vi "Open Front Panel.vi"(8 "Error In":errorcluster, 11 "Display Panel V3 in":refnum<class "Display Panel V3.lvclass">) -> (0 "Error Out":errorcluster, 3 "Display Panel V3 out":refnum<class "Display Panel V3.lvclass">)   [LabVIEW 2014, in "Display Panel.lvlib" / "Display Panel V3.lvclass"]
uses:
  Display Panel V3.lvclass
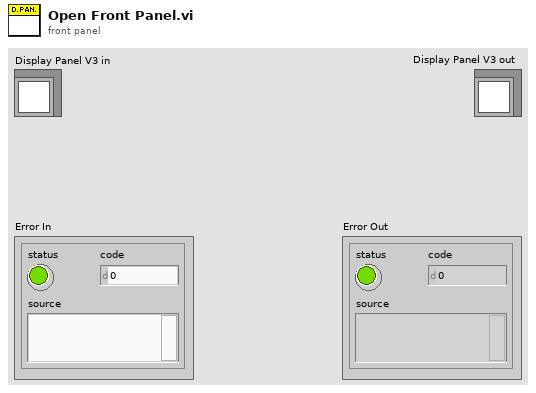
[diagram p1: front panel]
types:
  T1 = enum32{"Invalid", "Standard", "Closed", "Hidden", "Minimized", "Maximized"}
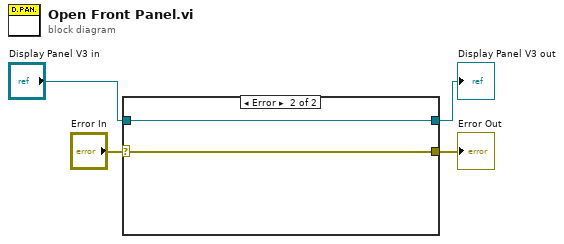
[diagram p0: block diagram]
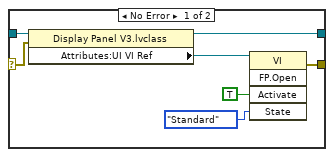
[diagram p2: hidden frame]
diagram:
  n1 = case shown="Error" "Error In" {
    selector: "Error In" -> [w10 w12]
    tunnel: "Display Panel V3 in" -> [w11 w13]
    tunnel: [w6 w12] -> w2
    tunnel: [w5 w13] -> w1
    frame No Error {
      n2 = property class="Display Panel V3.lvclass"(reference=w11, error in=w10) -> (reference out=w5:refnum<class "Display Panel V3.lvclass">, "Attributes:UI VI Ref"=w9:refnum<vi>)  [unwired: 1 out]
      n3 = invoke class="VI" method="FP.Open"(reference=w9, "Activate"=TRUE ("Activate?"), "State"=T1."Standard") -> (error out=w6:errorcluster)  [unwired: 2 in, 4 out]
    }
    frame Error {
    }
  }
  "Error Out" <- w2
  "Display Panel V3 out" <- w1
